vi "2.设置文件夹和名称.vi"(8 "error in":errorcluster, 9 "Name":string, 10 "BasePath":path, 11 "Module ID":i32=-1) -> (0 "error out":errorcluster, 3 "Module ID out":i32=-1)   [LabVIEW 2020, in "Log.lvlib"]
uses:
  Log.lvlib
  Log.lvlibp
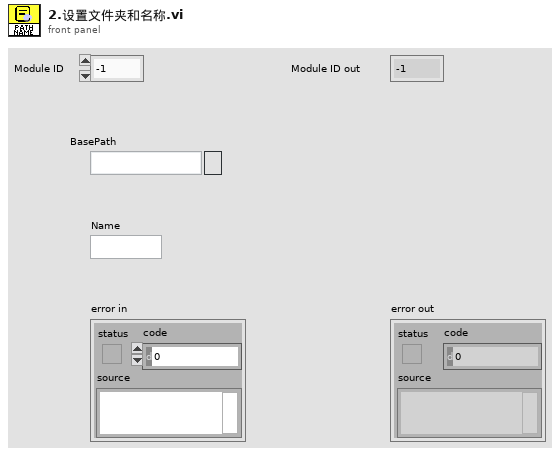
[diagram p1: front panel]
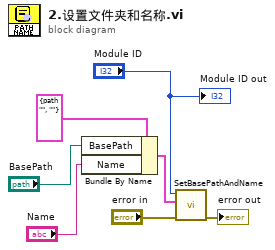
[diagram p0: block diagram]
diagram:
  n1 = Bundle By Name(cluster=cluster{"BasePath":path, "Name":string} {"BasePath"=path "", "Name"=""} ("PathAndName"), "BasePath"="BasePath", "Name"="Name") -> (w3:cluster{"BasePath":path, "Name":string})
  n2 = call "SetBasePathAndName.vi"("error in"="error in", "PathAndName"=w3, "Module ID"="Module ID") -> ("error out"=→"error out":errorcluster)  [unwired: 8 in]
  "Module ID out" <- "Module ID"
